vi "Do Request.vi"(7 "Processing In":refnum<class "Processing.lvclass">, 11 "History Data Controller in":refnum<class "History Data Controller.lvclass">) -> (0 "error out":errorcluster, 5 "Processing":refnum<class "Processing.lvclass">)   [LabVIEW 2020, in "VolatusHistorian.lvlib" / "History Data Controller.lvclass"]
doc: "A controller's main job is to respond to a request by generating a response. The response value must be specified by calling Set Response.vi on the Processing class that's passed through the VI otherwise an error will be generated.\n\nThere are several helpers available for common response types:\nGenerating HTML content programmatically - Create Basic Response.vi\nStreaming a file from disk - Create File Response.vi\nRedirecting the user to another URL - Create Redirect Response.vi\n\nFile responses are streamed in chunks and do not load the entire file into memory at once to send in the response which allows serving large files more efficiently."
uses:
  History Data Controller.lvclass
  lv-http-server/HTTP Server/Processing/Processing.lvclass
  History Data Controller.lvclass/History Data Controller.ctl
  lv-http-server/HTTP Server/Processing/Processing.lvclass/Processing.ctl
  lv-http-util/HTTP Utils/Request/Request.lvclass/Request.ctl
  lv-uri/URI/URI/URI.lvclass/URI.ctl
  Time Format.ctl
  Data Request.ctl
  History Data Value/Unix ns Data Value.lvclass
  History Data Value/Unix ns Data Value.lvclass/Unix ns Data Value.ctl
  Local Data Value/LV Dbl Data Value.lvclass
  Local Data Value/LV Dbl Data Value.lvclass/LV Dbl Data Value.ctl
  lv-uri/URI/URI/Path String.vi
  lv-http-util/HTTP Utils/Request/Request.lvclass
  lv-http-util/HTTP Utils/Response/Response.lvclass
  VolatusHistorian.lvlib
  lv-vecto/Vecto/Vecto.lvlib
  Volatus/MessageQ/MessageQ.lvclass
  lv-uri/URI/URI/URI.lvclass
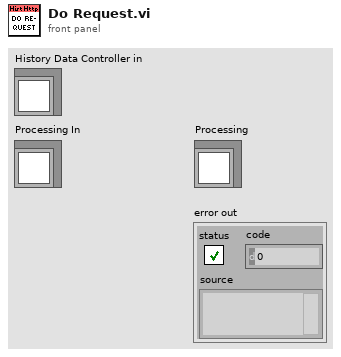
[diagram p1: front panel]
types:
  T1 = typedef "VolatusHistorian.lvlib/Time Format.ctl" = enum16{"unix_ns", "lv"}
  T2 = typedef "VolatusHistorian.lvlib/Data Request.ctl" = cluster{"Channels":string[], "Start Time":dbl, "End Time":dbl, "Time Format":T1}
  T3 = typedef "VolatusHistorian.lvlib/History Data (unix ns).ctl" = cluster{"Channels":T4[]}
  T4 = typedef "VolatusHistorian.lvlib/Channel History (unix ns).ctl" = cluster{"Name":string, "Unix_ns":i64[], "Data":dbl[]}
  T5 = typedef "VolatusHistorian.lvlib/History Data (LV Dbl).ctl" = cluster{"Channels":T6[]}
  T6 = typedef "VolatusHistorian.lvlib/Channel History (LV Dbl).ctl" = cluster{"Name":string, "Timestamps":dbl[], "Data":dbl[]}
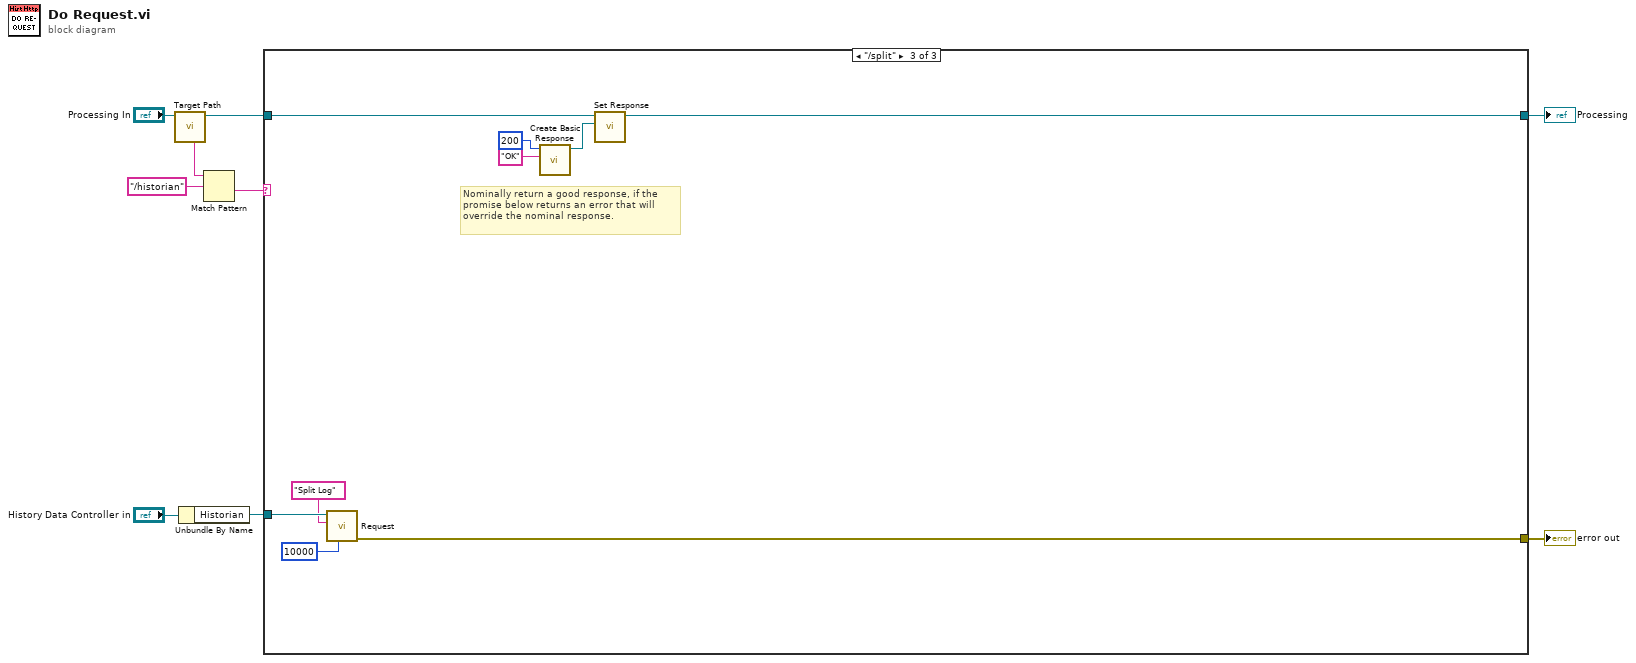
[diagram p0: block diagram]
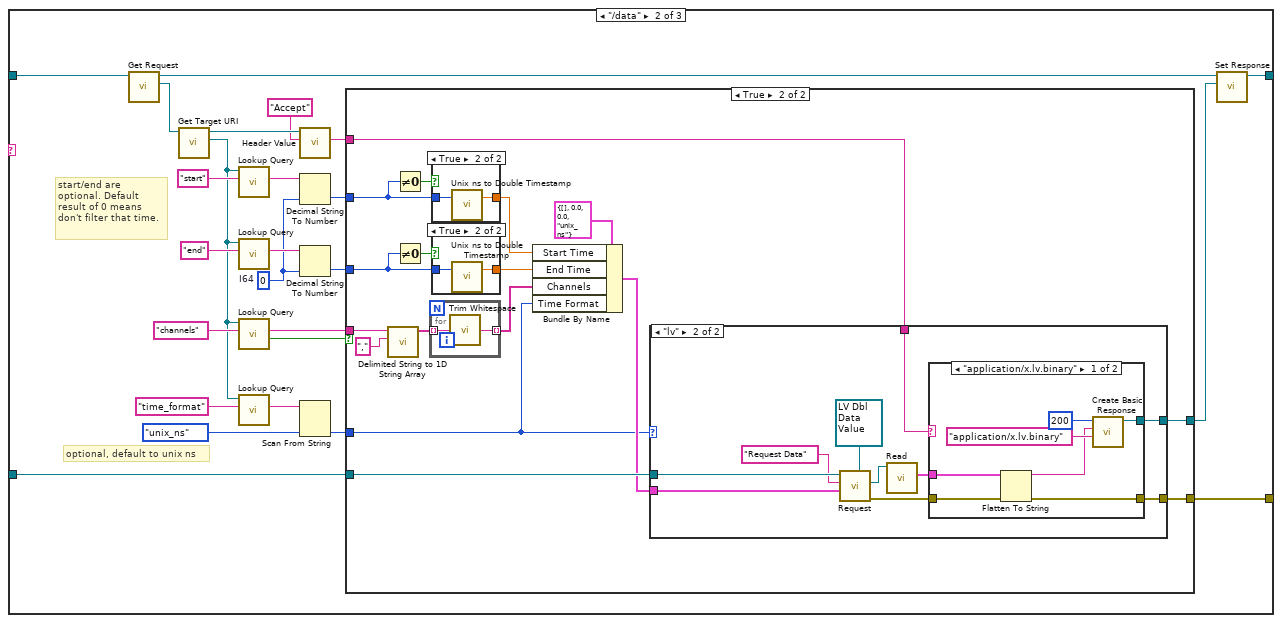
[diagram p3: hidden frame]
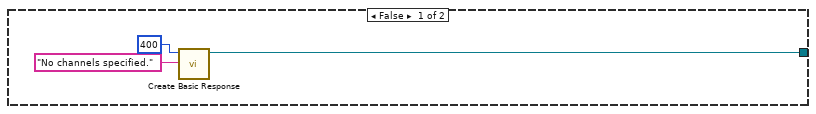
[diagram p4: hidden frame]
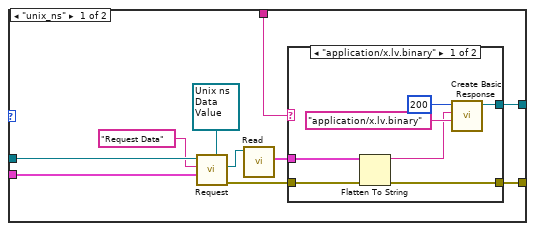
[diagram p5: hidden frame]
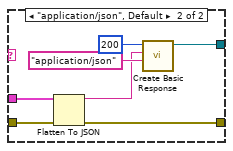
[diagram p6: hidden frame]
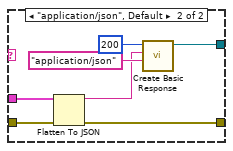
[diagram p7: hidden frame]
diagram:
  n1 = call "Target Path.vi"("Processing in"="Processing In") -> ("Processing out"=w5:refnum<class "Processing.lvclass">, "Target Path"=w9:string)  [unwired: 9 in]
  n2 = Unbundle By Name("History Data Controller in") -> ("Historian"=w3:refnum<class "MessageQ.lvclass">)
  n3 = Match Pattern(string=w9, regular expression="/historian") -> (after substring=w6:string)  [unwired: 1 in, 3 out]
  n4 = case shown="\"/split\"" w6 {
    tunnel: w5 -> [w10 w35 w112]
    tunnel: w3 -> [_ w21 w118]
    tunnel: [w10 w22 w110] -> w2
    tunnel: [_ w20 w115] -> w1
    frame Default {
    }
    frame "/data" {
      w24 = i64 0  # I64
      # "start/end are optional. Default result of 0 means don't filter that time."
      # "optional, default to unix ns"
      n5 = call "Get Request.vi"("Processing in"=w35) -> ("Request"=w34:refnum<class "Request.lvclass">, "Processing out"=w23:refnum<class "Processing.lvclass">)  [unwired: 9 in]
      n6 = call "Get Target URI.vi"("Request in"=w34) -> ("Target URI"=w18:refnum<class "URI.lvclass">, "Request out"=w13:refnum<class "Request.lvclass">)  [unwired: 8 in, 1 out]
      n7 = call "Lookup Query.vi"("Name"="start", "URI in"=w18) -> ("Value"=w30:string)  [unwired: 7 in, 2 out]
      n8 = call "Lookup Query.vi"("Name"="end", "URI in"=w18) -> ("Value"=w26:string)  [unwired: 7 in, 2 out]
      n9 = call "Lookup Query.vi"("Name"="channels", "URI in"=w18) -> ("Found"=w28:bool, "Value"=w29:string)  [unwired: 7 in, 1 out]
      n10 = call "Lookup Query.vi"("Name"="time_format", "URI in"=w18) -> ("Value"=w17:string)  [unwired: 7 in, 2 out]
      n11 = call "Header Value.vi"("Header"="Accept", "Request in"=w13) -> ("Value"=w11:string)  [unwired: 6 in, 3 out]
      n12 = Decimal String To Number(string=w30, default (0L)=w24) -> (number=w27:i64)  [unwired: 1 in, 1 out]
      n13 = Decimal String To Number(string=w26, default (0L)=w24) -> (number=w25:i64)  [unwired: 1 in, 1 out]
      n14 = Scan From String(input string=w17, default 1=Time_Format."unix_ns" ("Time Format")) -> (output 1=w15:T1)  [unwired: 3 in, 3 out]
      n15 = case shown="True" w28 {
        tunnel: w29 -> [_ w55]
        tunnel: w27 -> [_ w52]
        tunnel: w25 -> [_ w49]
        tunnel: w21 -> [_ w44]
        tunnel: [_ w42] -> w20
        tunnel: w15 -> [_ w39]
        tunnel: [w36 w41] -> w14
        tunnel: w11 -> [_ w40]
        frame False {
          n16 = call "Create Basic Response.vi"("Payload"="No channels specified.", "Status Code"=u16 400) -> ("Response out"=w36:refnum<class "Response.lvclass">)  [unwired: 8 in, 1 out]
        }
        frame True {
          n17 = call <vilib>:"Delimited String to 1D String Array.vi"("delimiter"=",", "delimited string"=w55) -> ("string array"=w53:string[])  [unwired: 9 in]
          n18 = Not Equal To 0?(x=w52) -> (x != 0?=w51:bool)
          n19 = Not Equal To 0?(x=w49) -> (x != 0?=w50:bool)
          n20 = for {
            tunnel: w53 -> [w109] mode=indexing
            tunnel: [w108] -> w46 mode=indexing
            n21 = call <vilib>:"Trim Whitespace.vi"("string"=w109) -> ("trimmed string"=w108:string)  [unwired: 1 in]
          }
          n22 = case shown="True" w51 {
            tunnel: w52 -> [_ w107]
            tunnel: [_ w106] -> w45
            frame False {
            }
            frame True {
              n23 = call "Unix ns to Double Timestamp.vi"("unix ns"=w107) -> ("Timestamp"=w106:dbl)  [unwired: 2 in]
            }
          }
          n24 = case shown="True" w50 {
            tunnel: w49 -> [_ w105]
            tunnel: [_ w104] -> w47
            frame False {
            }
            frame True {
              n25 = call "Unix ns to Double Timestamp.vi"("unix ns"=w105) -> ("Timestamp"=w104:dbl)  [unwired: 2 in]
            }
          }
          n26 = Bundle By Name(cluster=T2 {"Channels"=[], "Start Time"=0.0, "End Time"=0.0, "Time Format"=enum."unix_ns"} ("Data Request"), "Start Time"=w45, "End Time"=w47, "Channels"=w46, "Time Format"=w39) -> (w43:T2)
          n27 = case shown="\"lv\"" w39 {
            tunnel: w44 -> [w65 w89]
            tunnel: w43 -> [w63 w87]
            tunnel: [w58 w81] -> w42
            tunnel: [w57 w80] -> w41
            tunnel: w40 -> [w56 w82]
            frame "unix_ns" {
              n28 = call "Request.vi"("Response Type (None)"=refnum<class "Unix ns Data Value.lvclass"> refnum ("VolatusHistorian.lvlib:History Data Value.lvclass"), "Data"=w63, "ID"="Request Data", "MessageQ in"=w65) -> ("error out"=w59:errorcluster, "Response"=w61:refnum<class "Unix ns Data Value.lvclass">)  [unwired: 5 in, 1 out]
              n29 = call "Read.vi"("History Data Value in"=w61) -> ("Data"=w60:T3)  [unwired: 10 in]
              n30 = case shown="\"application/x.lv.binary\"" w56 {
                tunnel: w60 -> [w72 w79]
                tunnel: w59 -> [w71 w78]
                tunnel: [w70 w77] -> w58
                tunnel: [w67 w73] -> w57
                frame "application/x.lv.binary" {
                  n31 = Flatten To String(anything=w72, error in (no error)=w71) -> (data string=w66:string, error out=w70:errorcluster)  [unwired: 2 in, 1 out]
                  n32 = call "Create Basic Response.vi"("Content-Type (text/plain)"="application/x.lv.binary", "Payload"=w66, "Status Code"=u16 200) -> ("Response out"=w67:refnum<class "Response.lvclass">)  [unwired: 7 in, 1 out]
                }
                frame "application/json", Default {
                  n33 = Flatten To JSON(anything=w79, error in (no error)=w78) -> (JSON string=w74:string, 11:w77:errorcluster)  [unwired: 1 in]
                  n34 = call "Create Basic Response.vi"("Content-Type (text/plain)"="application/json", "Payload"=w74, "Status Code"=u16 200) -> ("Response out"=w73:refnum<class "Response.lvclass">)  [unwired: 7 in, 1 out]
                }
              }
            }
            frame "lv" {
              n35 = call "Request.vi"("Response Type (None)"=refnum<class "LV Dbl Data Value.lvclass"> refnum ("VolatusHistorian.lvlib:Local Data Value.lvclass"), "Data"=w87, "ID"="Request Data", "MessageQ in"=w89) -> ("error out"=w84:errorcluster, "Response"=w85:refnum<class "LV Dbl Data Value.lvclass">)  [unwired: 5 in, 1 out]
              n36 = call "Read.vi"("Local Data Value in"=w85) -> ("Data"=w83:T5)  [unwired: 10 in]
              n37 = case shown="\"application/x.lv.binary\"" w82 {
                tunnel: w83 -> [w96 w103]
                tunnel: w84 -> [w95 w102]
                tunnel: [w94 w101] -> w81
                tunnel: [w91 w97] -> w80
                frame "application/x.lv.binary" {
                  n38 = Flatten To String(anything=w96, error in (no error)=w95) -> (data string=w90:string, error out=w94:errorcluster)  [unwired: 2 in, 1 out]
                  n39 = call "Create Basic Response.vi"("Content-Type (text/plain)"="application/x.lv.binary", "Payload"=w90, "Status Code"=u16 200) -> ("Response out"=w91:refnum<class "Response.lvclass">)  [unwired: 7 in, 1 out]
                }
                frame "application/json", Default {
                  n40 = Flatten To JSON(anything=w103, error in (no error)=w102) -> (JSON string=w98:string, 11:w101:errorcluster)  [unwired: 1 in]
                  n41 = call "Create Basic Response.vi"("Content-Type (text/plain)"="application/json", "Payload"=w98, "Status Code"=u16 200) -> ("Response out"=w97:refnum<class "Response.lvclass">)  [unwired: 7 in, 1 out]
                }
              }
            }
          }
        }
      }
      n42 = call "Set Response.vi"("Response"=w14, "Processing in"=w23) -> ("Processing out"=w22:refnum<class "Processing.lvclass">)  [unwired: 9 in]
    }
    frame "/split" {
      # "Nominally return a good response, if the promise below returns an error that will override the nominal response."
      n43 = call "Request.vi"("Timeout ms (1000)"=10000, "ID"="Split Log", "MessageQ in"=w118) -> ("error out"=w115:errorcluster)  [unwired: 6 in, 2 out]
      n44 = call "Create Basic Response.vi"("Payload"="OK", "Status Code"=u16 200) -> ("Response out"=w111:refnum<class "Response.lvclass">)  [unwired: 8 in, 1 out]
      n45 = call "Set Response.vi"("Response"=w111, "Processing in"=w112) -> ("Processing out"=w110:refnum<class "Processing.lvclass">)  [unwired: 9 in]
    }
  }
  "error out" <- w1
  "Processing" <- w2
